vi "commandCompleted.vi"(8 "error in (no error)":errorcluster, 11 "ElectrometerController in":refnum<class "ElectrometerController.lvclass">) -> (0 "error out":errorcluster, 3 "ElectrometerController out":refnum<class "ElectrometerController.lvclass">)   [LabVIEW 2016, in "ElectrometerController.lvclass"]
uses:
  ElectrometerController.lvclass
  ts_electrometeruserevents/Typedefs/CommandValue.ctl
  ElectrometerController.lvclass/ElectrometerController.ctl
  ts_electrometeruserevents/PubSubDataEvent/PubSubDataEvent.lvclass
  ts_electrometeruserevents/Typedefs/ElectrometerTypedefs.lvlib
  InternalCommandId/InternalCommandId.lvclass
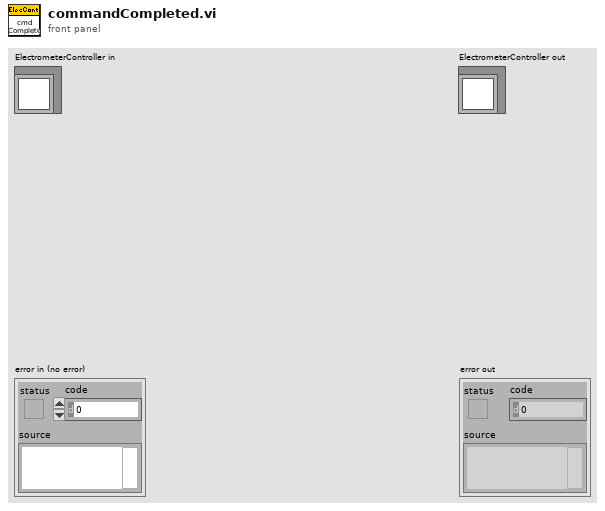
[diagram p1: front panel]
types:
  T1 = typedef "ElectrometerTypedefs.lvlib/CommandValue.ctl" = enum16{"ClearError", "Disable", "Enable", "Exit", "GoToStandby", "OnHeartbeat", "OnIncomingMessagingError", "OnInterrupt", "Start", "SetDigitalFilter", "StartScan", "StartScanDt", "StartScanReachIntensity", "StopScan", "SetIntegrationTime", "PerformZeroCalib", "SetRange", "SetMode", "Power"}
  T2 = cluster{"error":i32, "result":string, "ack":i32, "cmdSeqNum":i32, "CommandValue":T1}
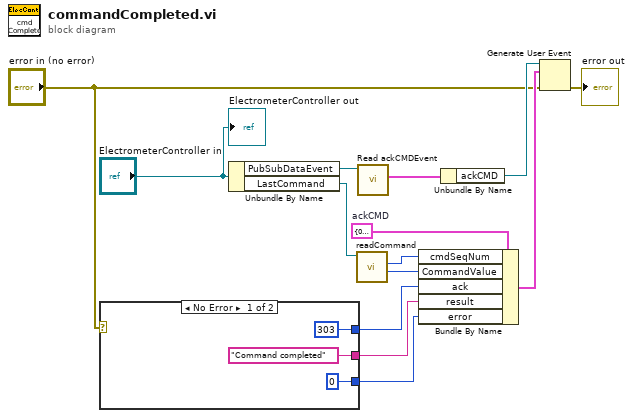
[diagram p0: block diagram]
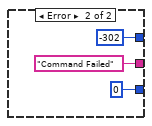
[diagram p2: hidden frame]
diagram:
  w12 = T2 {"error"=0, "result"="", "ack"=0, "cmdSeqNum"=0, "CommandValue"=enum."ClearError"}  # ackCMD
  n1 = case shown="No Error" "error in (no error)" {
    tunnel: [0 ("error") 0 ("error")] -> w5
    tunnel: ["Command completed" ("result") "Command Failed" ("result")] -> w6
    tunnel: [303 ("ack") -302 ("ack")] -> w7
    frame No Error {
    }
    frame Error {
    }
  }
  n2 = Unbundle By Name("ElectrometerController in") -> ("PubSubDataEvent"=w9:refnum<class "PubSubDataEvent.lvclass">, "LastCommand"=w3:refnum<class "InternalCommandId.lvclass">)
  n3 = call "readCommand.vi"("InternalCommandId in"=w3) -> ("CommandValue"=w1:T1, "CommandID"=w2:i32)  [unwired: 7 in, 2 out]
  n4 = call-dynamic "Read ackCMDEvent.vi"("PubSubDataEvent in"=w9) -> ("ackCMDEvent"=w13:cluster{"ackCMD":refnum<user-event>})  [unwired: 8 in, 2 out]
  n5 = Bundle By Name(cluster=w12, "cmdSeqNum"=w2, "CommandValue"=w1, "ack"=w7, "result"=w6, "error"=w5) -> (w11:T2)
  n6 = Unbundle By Name(w13) -> ("ackCMD"=w14:refnum<user-event>)
  n7 = Generate User Event(user event=w14, event data cluster=w11, error in="error in (no error)") -> (error out=→"error out":errorcluster)  [unwired: 1 in, 1 out]
  "ElectrometerController out" <- "ElectrometerController in"
